vi "Pre Launch Init.vi"(11 "Iterator Actor in":refnum<class "Iterator NR Actor.lvclass">) -> (0 "error out":errorcluster, 3 "Iterator Actor out":refnum<class "Iterator NR Actor.lvclass">)   [LabVIEW 2023, in "Iterator Actor.lvlib" / "Iterator NR Actor.lvclass"]
doc: "(<B>Filename</B>: Actor Framework.lvlib:Actor.lvclass:Pre Launch Init.vi)\n\nDefines behavior that occurs after the Launch Nested Actor method is invoked but before the actor's Actor Core method begins running.\n\nBy default, this method does nothing. A descendant class may override it to define behavior."
uses:
  Iterator NR Actor.lvclass
  Iterator NR Actor.lvclass/Iterator NR Actor.ctl
  Abstract Iterator Actor/Abstract Iterator Actor.lvclass
  <userlib>/_OpenG.lib/error/error.llb/openg_error.lvlib
  Iterator NR Actor Messages/Request Iteration Notification Msg/Request Iteration Notification Msg.lvclass
  <vilib>/ActorFramework/Actor/Actor.lvclass
  C:/Projects/Iterator Actor/Abstract Iterator Actor/Abstract Iterator Actor.lvclass
  C:/Program Files/National Instruments/LabVIEW 2023/vi.lib/LS Instruments AG/Async Methods Actor/Async Methods Actor/Async Methods Actor/Async Methods Actor.lvclass
  C:/Program Files/National Instruments/LabVIEW 2023/vi.lib/ActorFramework/Actor/Actor.lvclass
  C:/Projects/Iterator Actor/Iterator NR Actor/Iterator NR Actor Folder/Iterator NR Actor.lvclass
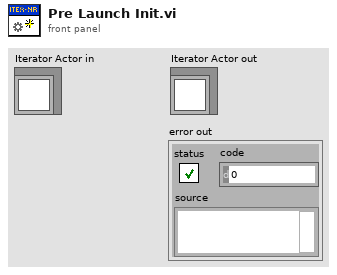
[diagram p1: front panel]
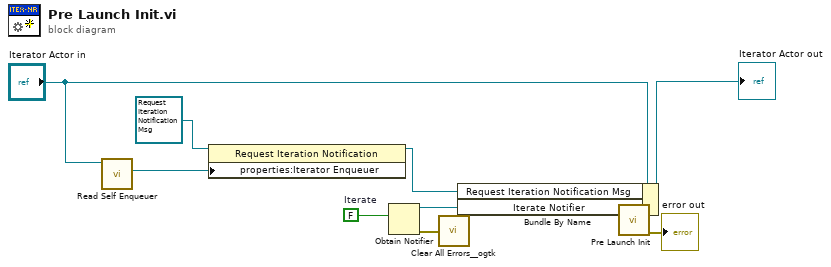
[diagram p0: block diagram]
diagram:
  w7 = FALSE  # Iterate
  n1 = call <vilib>:"Read Self Enqueuer.vi"("Actor"="Iterator Actor in") -> ("Self Enqueuer"=w1:refnum<class "Message Enqueuer.lvclass">)  [unwired: 10 in]
  n2 = property class="Request Iteration Notification "(reference=refnum<class "Request Iteration Notification Msg.lvclass"> refnum ("Iterator Actor.lvlib:Request Iteration Notification Msg.lvclass"), "properties:Iterator Enqueuer"=w1) -> (reference out=w2:refnum<class "Request Iteration Notification Msg.lvclass">)  [unwired: 1 in, 1 out]
  n3 = Obtain Notifier(notification data type=w7) -> (notifier out=w6:refnum<notifier>, error out=w5:errorcluster)  [unwired: 3 in, 1 out]
  n4 = call <userlib>:"Clear All Errors__ogtk.vi"("Error In"=w5) -> ()  [unwired: 3 in, 1 out]
  n5 = Bundle By Name(cluster="Iterator Actor in", "Request Iteration Notification Msg"=w2, "Iterate Notifier"=w6) -> (w8:refnum<class "Iterator NR Actor.lvclass">)
  n6 = call-parent "Pre Launch Init.vi"("Iterator Actor in"=w8) -> ("error out"=→"error out":errorcluster, "Iterator Actor out"=→"Iterator Actor out":refnum<class "Iterator NR Actor.lvclass">)  [unwired: 9 in]
